vi "Get SMO Name.vi"(8 "error in (no error)":errorcluster, 11 "Instrument in":refnum<class "Instrument.lvclass">) -> (0 "error out":errorcluster, 1 "SMO Vendor":string, 2 "SMO Name":string, 3 "Instrument out":refnum<class "Instrument.lvclass">)   [LabVIEW 2019, in "Instrument.lvclass"]
doc: "Override this VI to return the name of your Instrument"
uses:
  Instrument.lvclass
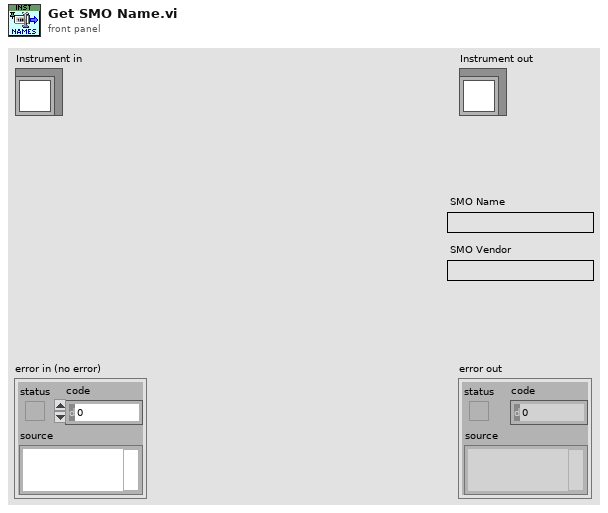
[diagram p1: front panel]
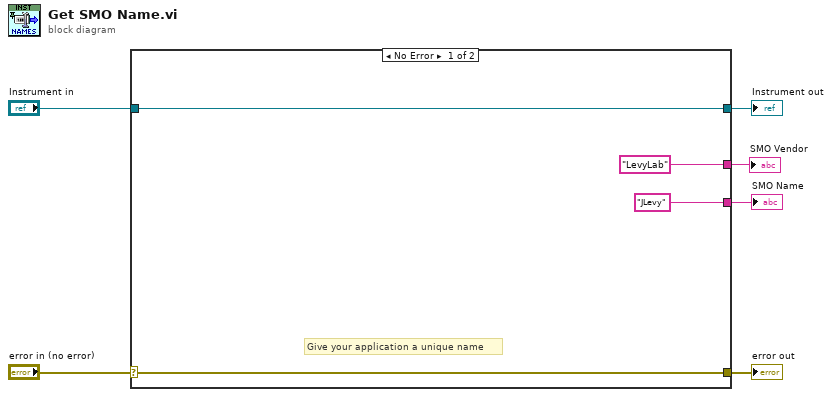
[diagram p0: block diagram]
diagram:
  n1 = case shown="No Error" "error in (no error)" {
    selector: "error in (no error)" -> [w9 w12]
    tunnel: [w9 w12] -> w5
    tunnel: [w10 w11] -> w3
    tunnel: "Instrument in" -> [w10 w11]
    tunnel: ["JLevy" ("SMO Name") _] -> w2
    tunnel: ["LevyLab" ("SMO Vendor") _] -> w1
    frame No Error {
      # "Give your application a unique name"
    }
    frame Error {
    }
  }
  "error out" <- w5
  "Instrument out" <- w3
  "SMO Name" <- w2
  "SMO Vendor" <- w1
